vi "Draw Tree and set expand settings.vi"(8 "error in":errorcluster, 10 "Tree Map In":T1, 11 "TreeControl in":refnum<vi>) -> (0 "error out":errorcluster)   [LabVIEW 2019, in "Panther Dashboard.lvlib"]
uses:
  Panther Dashboard.lvlib
  <vilib>/National Instruments/Tree Map/Tree Map Data.ctl
  <vilib>/National Instruments/Tree Map/API/List Roots.vi
  <vilib>/National Instruments/Tree Map/Utility/Into Tree Control Items.vi
  <vilib>/National Instruments/Tree Map/Tree Map.lvlib
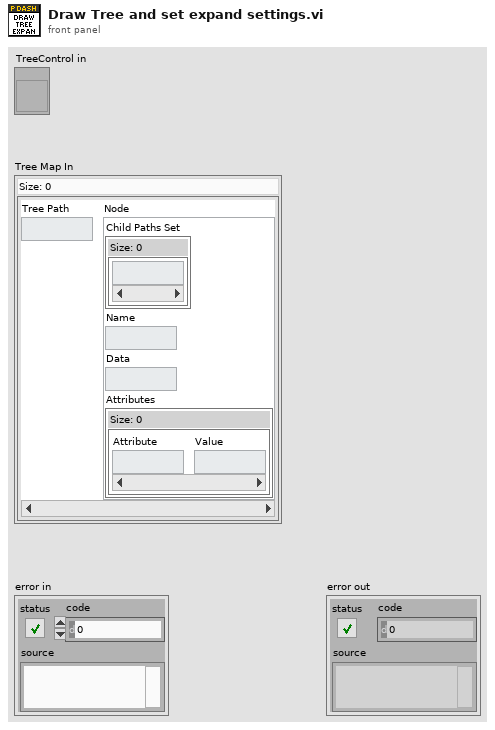
[diagram p1: front panel]
types:
  T1 = typedef "Tree Map.lvlib/Tree Map Data.ctl" = map{string, cluster{"Child Paths Set":set{string}, "Name":string, "Data":string, "Attributes":map{string, string}}}
  T2 = cluster{"Left Cell String":string, "Child Text":string[], "Child Tag":string, "Item Indent":i32, "Child Only?":bool, "Glyph Index":i32}[]
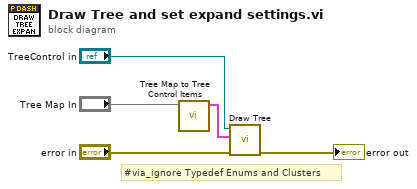
[diagram p0: block diagram]
diagram:
  # "#via_ignore Typedef Enums and Clusters"
  n1 = call <vilib>:"Tree Map to Tree Control Items.vi"("Tree Map In"="Tree Map In") -> ("Tree Control Items"=w2:T2)  [unwired: 10 in]
  n2 = call "Draw Tree.vi"("error in"="error in", "Tree Control Items"=w2, "TreeControl in"="TreeControl in") -> ("error out"=→"error out":errorcluster)  [unwired: 7 in, 1 out]
